vi "sub1.vi"(9 "Part References.Parse State Queue":refnum<vi>, 10 "regular expression":string, 11 "Array":T1(array[cluster])) -> (3 "Tunnel out":refnum<vi>)   [LabVIEW 2017, in "CSM-Helper.lvclass"]
doc: "### sub1.vi\n\n-- <b>Controls</b> --\n- <b>Part References.Parse State Queue</b>:\n- <b>regular expression</b>:\n- <b>Array</b>:\n\n-- <b>Indicators</b> --\n- <b>Tunnel out</b>:"
uses:
  CSM-Helper.lvclass
  Utility/_Support/Terminals.llb/csmHelper-Terminals.lvlib
panel:
  # "Connector Pane"
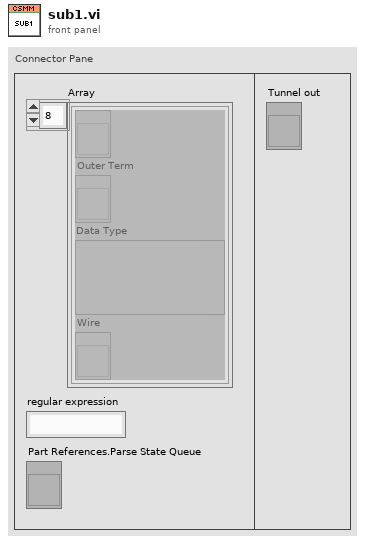
[diagram p1: front panel]
types:
  T1 = cluster{refnum<vi>, "Outer Term":refnum<vi>, "Data Type":variant, "Wire":refnum<vi>}[]
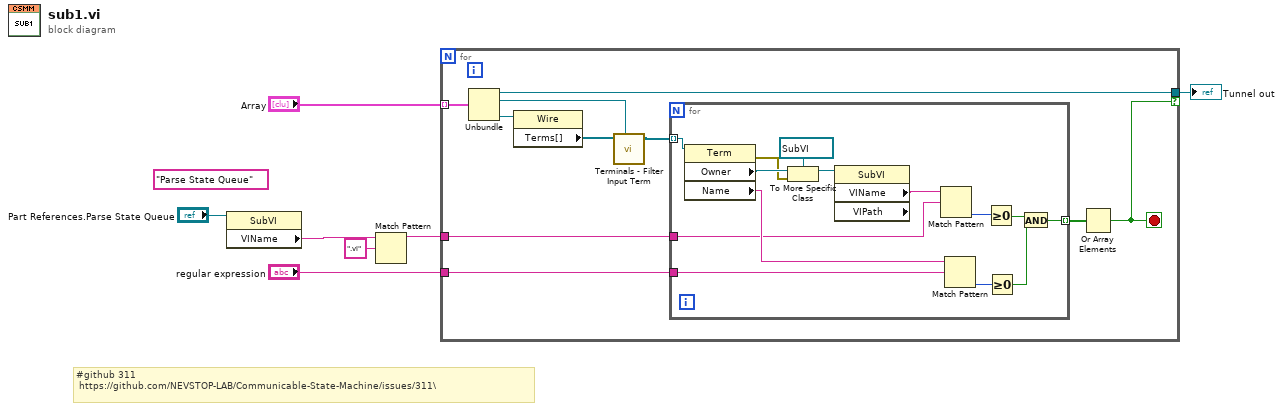
[diagram p0: block diagram]
diagram:
  (unwired) "Parse State Queue" ("regular expression")
  # "#github 311\n https://github.com/NEVSTOP-LAB/Communicable-State-Machine/issues/311\\"
  n1 = property class="SubVI"(reference="Part References.Parse State Queue") -> ("VIName"=w3:string)  [unwired: 1 in, 2 out]
  n2 = Match Pattern(string=w3, regular expression=".vi") -> (before substring=w1:string)  [unwired: 1 in, 3 out]
  n3 = for {
    tunnel: "Array" -> [w17] mode=indexing
    tunnel: [w15] -> w6 if=w12
    tunnel: "regular expression" -> [w13]
    tunnel: w1 -> [w8]
    stop <- w12 stop-if-true
    n4 = Unbundle(w17) -> (w15:refnum<vi>, "Outer Term"=w9:refnum<vi>, "Wire"=w16:refnum<vi>)  [unwired: 1 out]
    n5 = property class="Wire"(reference=w16) -> ("Terms[]"=w11:refnum<vi>[])  [unwired: 1 in, 2 out]
    n6 = call "Terminals - Filter Input Term.vi"("InnerTerminal in"=w9, "Wire.Terms[] in"=w11) -> ("Wire.Terms[] out"=w10:refnum<vi>[])  [unwired: 9 in]
    n7 = for {
      tunnel: [w21] -> w14 mode=indexing
      tunnel: w13 -> [w20]
      tunnel: w10 -> [w19] mode=indexing
      tunnel: w8 -> [w18]
      n8 = property class="Term"(reference=w19) -> (error out=w29:errorcluster, "Owner"=w31:refnum<vi>, "Name"=w26:string)  [unwired: 1 in, 1 out]
      n9 = To More Specific Class(target class=refnum<vi> refnum ("Parse State Queue"), reference=w31, error in=w29) -> (specific class reference=w28:refnum<vi>)  [unwired: 1 out]
      n10 = property class="SubVI" props=["VIName", "VIPath"](reference=w28) -> ("VIName"=w27:string)  [unwired: 1 in, 3 out]
      n11 = Match Pattern(string=w27, regular expression=w18) -> (offset past match=w25:i32)  [unwired: 1 in, 3 out]
      n12 = Match Pattern(string=w26, regular expression=w20) -> (offset past match=w24:i32)  [unwired: 1 in, 3 out]
      n13 = Greater Or Equal To 0?(x=w25) -> (x >= 0?=w23:bool)
      n14 = Greater Or Equal To 0?(x=w24) -> (x >= 0?=w22:bool)
      n15 = And(x=w23, y=w22) -> (x .and. y?=w21:bool)
    }
    n16 = Or Array Elements(Boolean array=w14) -> (logical OR=w12:bool)
  }
  "Tunnel out" <- w6
